vi "TEST Variant To Registry.vi"() -> ()   [LabVIEW 2013, in "Carya Config.lvclass"]
doc: "Copyright 2018, Carya Automatisering, Wiebe Walstra."
uses:
  Carya Config.lvclass
  CConfig Variant Accessor/CConfig Variant Accessor.lvclass
panel:
  out "data":T1
  out "error out":errorcluster
  out "String":string
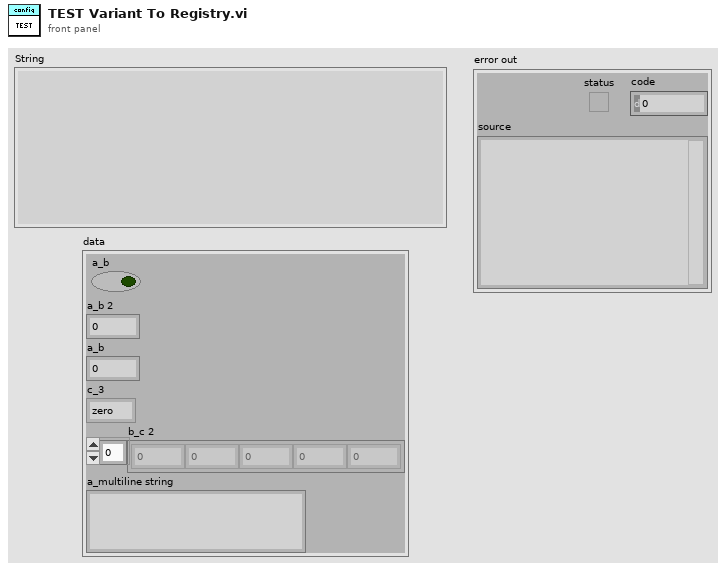
[diagram p1: front panel]
types:
  T1 = cluster{"a_b":bool, "a_b 2":i32, "a_b":csg, "c_3":enum16{"zero", "one", "two"}, "b_c 2":sgl[], "a_multiline string":string}
  T2 = cluster{"a_br":bool, "a_b 2":i32, "a_c":csg, "c_3":enum16{"zero", "one", "two"}, "b_c 2":sgl[], "a_multiline string":string}
  T3 = cluster{"a_b":i32, "a_b 2":i32, "a_c":csg, "c_3":enum16{"zero", "one", "two"}, "b_c 2":sgl[], "w_w":path[], "a_multiline string":string}
  T4 = cluster{"a_q":i32[], cluster{"a_b":i32, "a_b 2":i32, "a_c":csg, "c_3":enum16{"zero", "one", "two"}, "b_c 2":sgl[], "w_w":path[], "a_multiline string":string}}
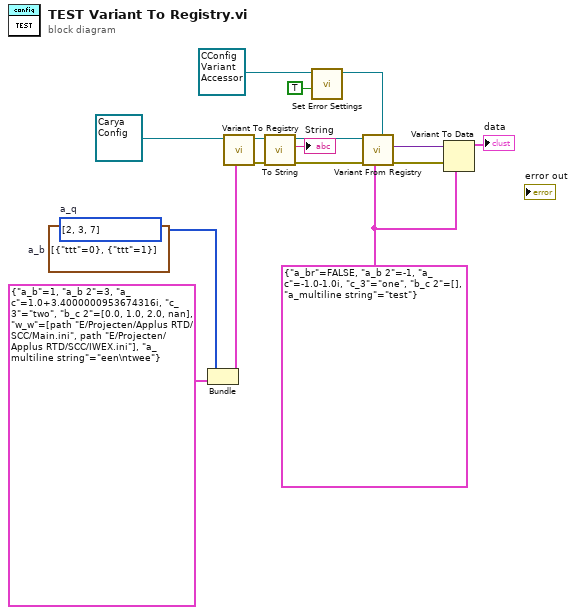
[diagram p0: block diagram]
diagram:
  w4 = T2 {"a_br"=FALSE, "a_b 2"=-1, "a_c"=-1.0-1.0i, "c_3"=enum."one", "b_c 2"=[], "a_multiline string"="test"}
  (unwired) cluster{"ttt":i32}[] [{"ttt"=0}, {"ttt"=1}]  # a_b
  w10 = i32[] [2, 3, 7]  # a_q
  n1 = Bundle("a_q"=w10, T3 {"a_b"=1, "a_b 2"=3, "a_c"=1.0+3.4i, "c_3"=enum."two", "b_c 2"=[0.0, 1.0, 2.0, nan], "w_w"=[path "E:/Projecten/Applus RTD/SCC/Main.ini", path "E:/Projecten/Applus RTD/SCC/IWEX.ini"], "a_multiline string"="een\ntwee"}) -> (w12:T4)  [unwired: 1 in]
  n2 = call "Variant To Registry.vi"("Variant"=w12, "Carya Config in"=refnum<class "Carya Config.lvclass"> refnum) -> ("error out"=w3:errorcluster, "Carya Config out"=w16:refnum<class "Carya Config.lvclass">)  [unwired: 6 in, 2 out]
  n3 = call-dynamic "To String.vi"("error in (no error)"=w3, "Carya Config in"=w16) -> ("error out"=w2:errorcluster, "String"=→"String":string, "Carya Config out"=w14:refnum<class "Carya Config.lvclass">)  [unwired: 7 in]
  n4 = call "Set Error Settings.vi"("Key not found error [F]"=TRUE ("Key not found error [T]"), "CConfig Variant Accessor in"=refnum<class "CConfig Variant Accessor.lvclass"> refnum) -> ("CConfig Variant Accessor out"=w6:refnum<class "CConfig Variant Accessor.lvclass">)  [unwired: 8 in, 1 out]
  n5 = call "Variant From Registry.vi"("Registry Variant Accessor in"=w6, "Variant"=w4, "error in (no error)"=w2, "Carya Config in"=w14) -> ("error out"=w1:errorcluster, "Variant"=w9:variant)  [unwired: 4 in, 2 out]
  n6 = Variant To Data(error in=w1, type=w4, Variant=w9) -> (data=→"data":T2)  [unwired: 1 out]
